vi "Actor Core.vi"(8 "error in":errorcluster, 11 "Main_Control in":refnum<class "Main_Control.lvclass">) -> (0 "error out":errorcluster, 3 "Actor out":refnum<class "Actor.lvclass">)   [LabVIEW 2021, in "Main_Control.lvlib" / "Main_Control.lvclass"]
doc: "(<B>Filename</B>: Actor Framework.lvlib:Actor.lvclass:Actor Core.vi)\n\nReceives messages to the actor, reacts to them, and initiates any error handling that may shut the actor down.\n\nDescendant classes may override this VI to append parallel tasks for the actor to complete while it handles messages. Overrides use the Call Parent Method node."
uses:
  Main_Control.lvclass
  C:/Program Files (x86)/National Instruments/LabVIEW 2021/vi.lib/ActorFramework/Actor/Actor.lvclass
  <vilib>/ActorFramework/Actor/Actor.lvclass
  NI/NI/NI.lvclass
  Camera/Camera/Camera.lvclass
  Utilities/RWC_Actions.ctl
  <vilib>/ActorFramework/Actor/Actor.lvclass/Actor.ctl
  <vilib>/ActorFramework/Message Enqueuer/Message Enqueuer.lvclass/Message Enqueuer.ctl
  Main_Control.lvclass/Main_Control.ctl
  Camera/Camera/Cam task parameters.ctl
  NI/NI/NI task parameters.ctl
  Camera/Camera Messages/Cam prepare task Msg/Cam prepare task Msg.lvclass/Cam prepare task Msg.ctl
  NI/NI Messages/NI prepare task Msg/NI prepare task Msg.lvclass/NI prepare task Msg.ctl
  <vilib>/ActorFramework/Message Enqueuer/Init from Existing Queue.vi
  <vilib>/ActorFramework/Message Enqueuer/Enqueue.vi
  NI/NI Messages/NI start task Msg/NI start task Msg.lvclass
  C:/Program Files (x86)/National Instruments/LabVIEW 2021/vi.lib/ActorFramework/Message/Message.lvclass
  <vilib>/ActorFramework/Stop Msg/Stop Msg.lvclass
  Camera/Camera Messages/Cam prepare task Msg/Cam prepare task Msg.lvclass
  NI/NI Messages/NI prepare task Msg/NI prepare task Msg.lvclass
  NI/NI Messages/NI stop task Msg/NI stop task Msg.lvclass
  <vilib>/ActorFramework/Message Priority Queue/Priority Enqueue.vi
  <vilib>/ActorFramework/Message Enqueuer/Message Enqueuer.lvclass
panel:
  out "time remain":dbl
  in  "Auto":bool
  out "Cam ready":bool
  out "NI ready":bool
  out "Cam":bool
  out "NI":bool
  in  "frame#":dbl=-1.0
  in  "save folder":path=path "D:/zyj workspace/SRIV/Temp File"
  in  "laser option":bool[](array[boolean])=[TRUE, FALSE, TRUE, FALSE]
  in  "buffer page #":dbl=20.0
  in  "flyback line #":dbl=400.0
  in  "camera H":dbl=8.0
  in  "camera W":dbl=768.0
  in  "exposure time":dbl=0.000107 min=1.7e-05 max=10.0
  in  "Update":bool
  in  "Acquire":bool
  out "auto start interval limit":dbl
  out "frame rate":dbl
  in  "laser all on?":bool
  in  "z offset":dbl
  in  "auto interval":dbl
  in  "z scan #":dbl=20.0
  in  "z step size":dbl=0.066
  in  "y pixel size":dbl=0.00059
  in  "y line #":dbl=9600.0
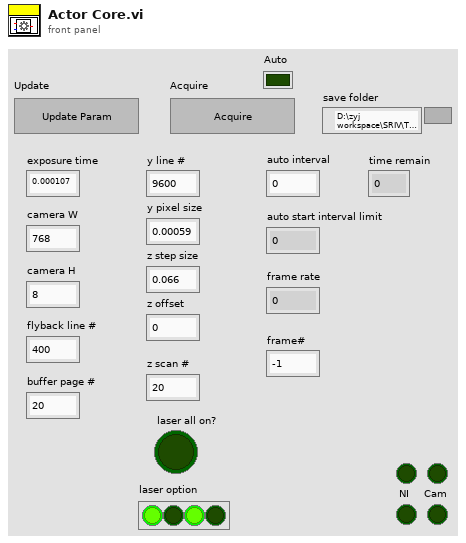
[diagram p1: front panel]
types:
  T1 = typedef "RWC_Actions.ctl" = enum16{"Read", "Write", "Read and Create"}
  T2 = typedef "NI.lvlib/NI.lvclass/NI task parameters.ctl" = cluster{"exposure time":dbl, "camera H":dbl, "y line #":dbl, "flyback line #":dbl, "y pixel size":dbl, "z scan #":dbl, "z step size":dbl, "z offset":dbl, "laser all on?":bool, "laser option":bool[]}
  T3 = typedef "Camera.lvlib/Camera.lvclass/Cam task parameters.ctl" = cluster{"exposure time":dbl, "camera W":dbl, "camera H":dbl, "y line #":dbl, "flyback line #":dbl, "buffer page#":dbl, "frame#":dbl}
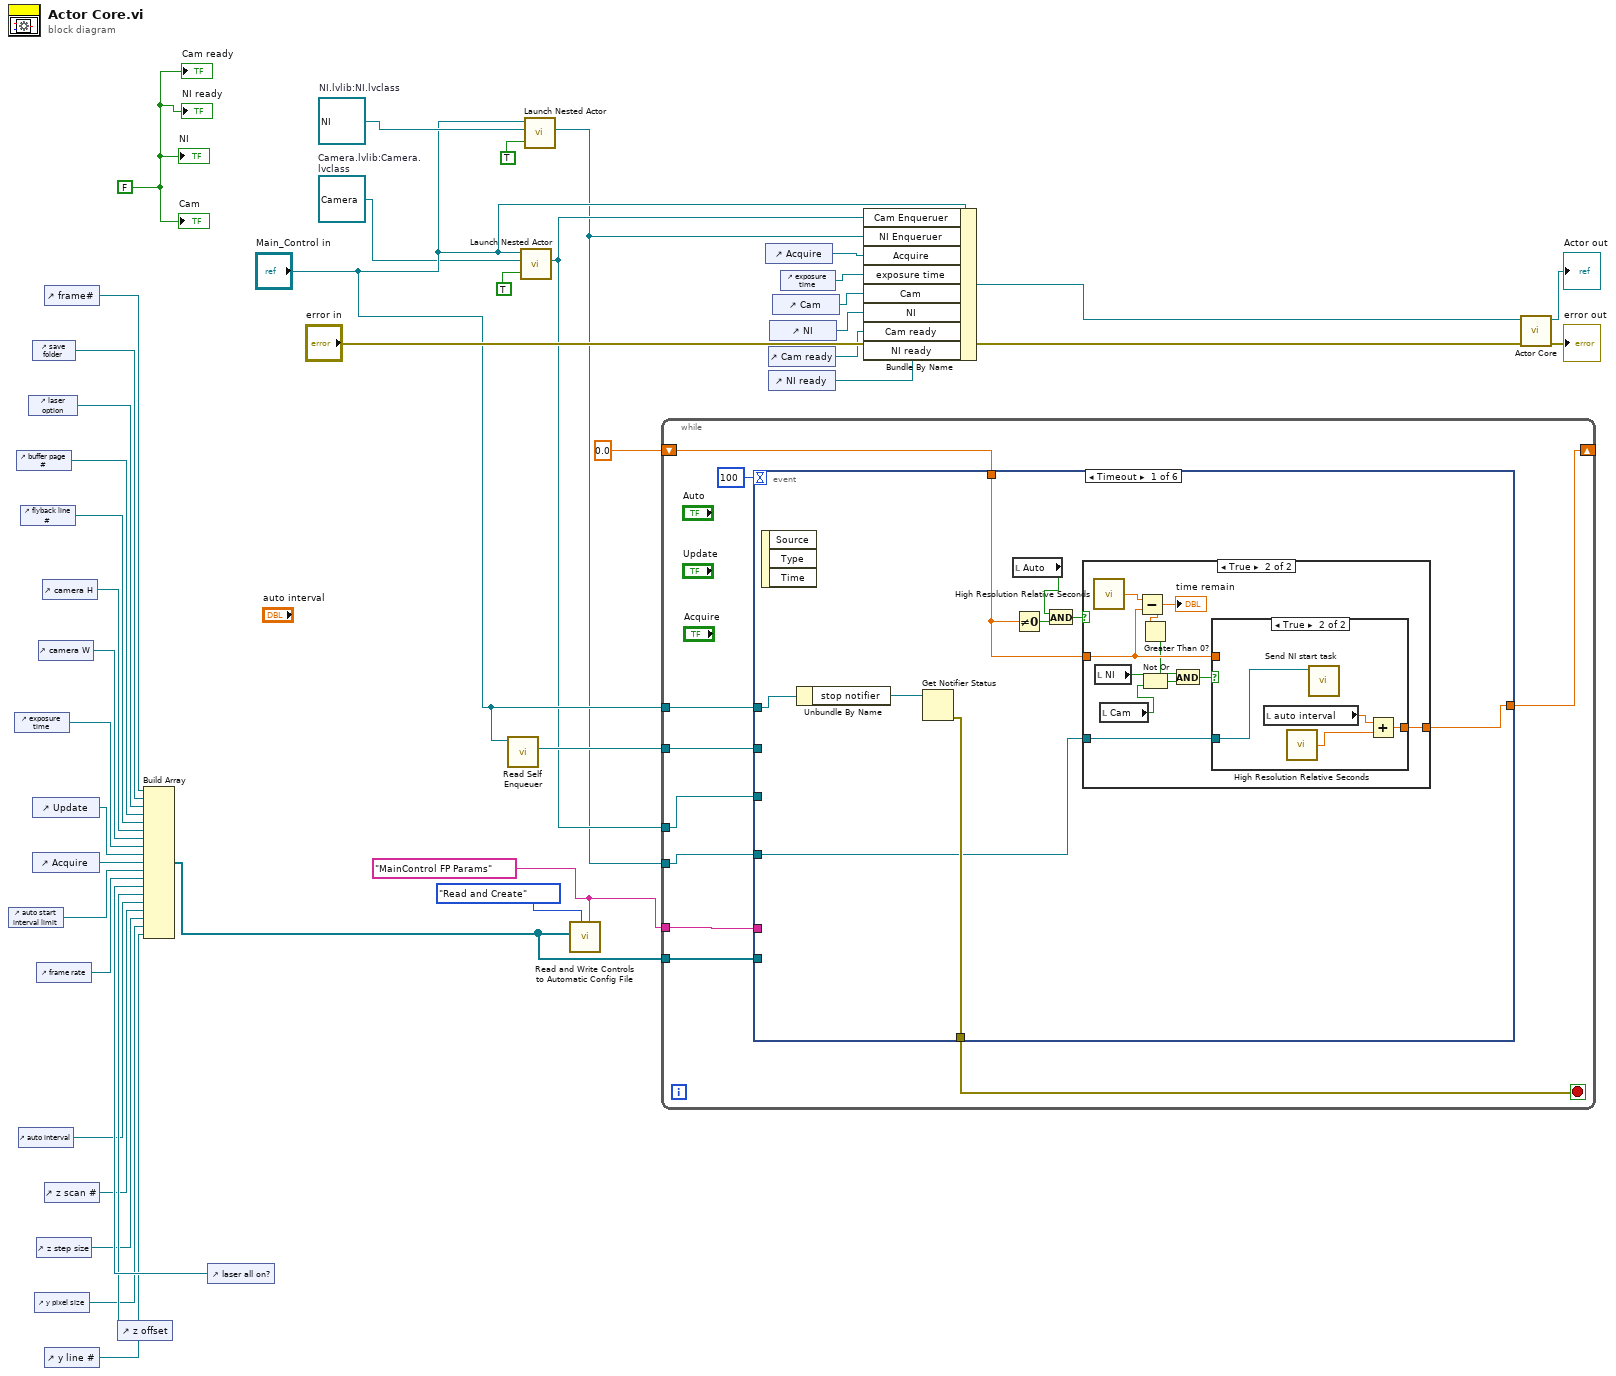
[diagram p0: block diagram]
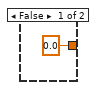
[diagram p2: hidden frame]
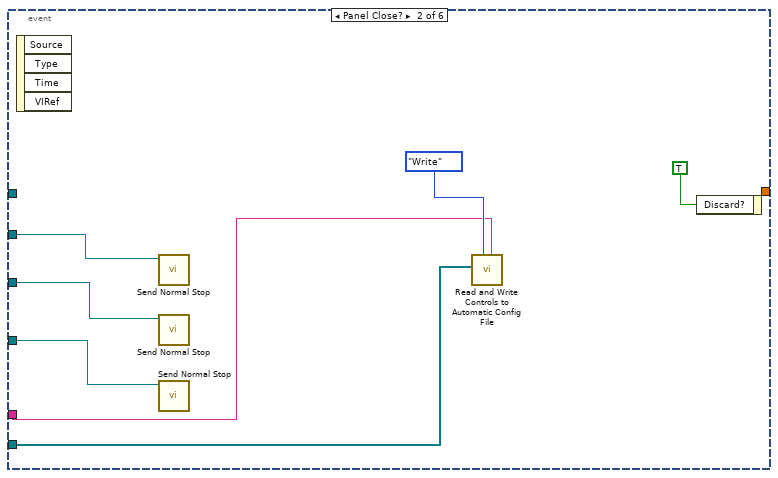
[diagram p4: hidden frame]
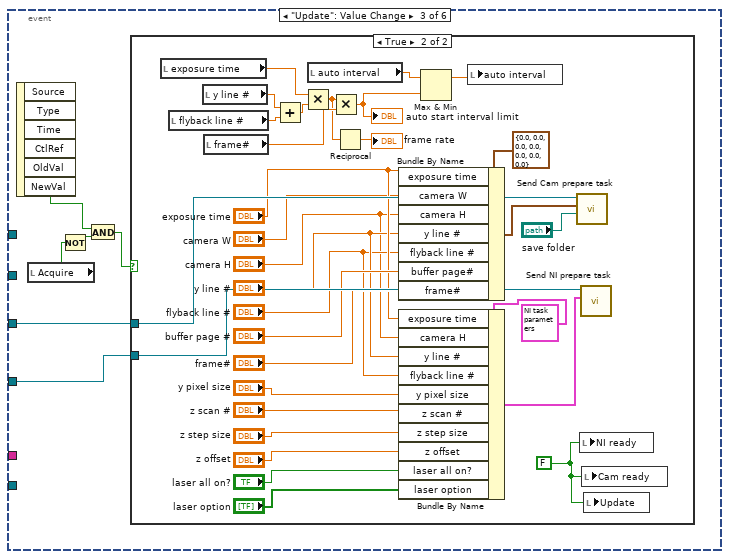
[diagram p5: hidden frame]
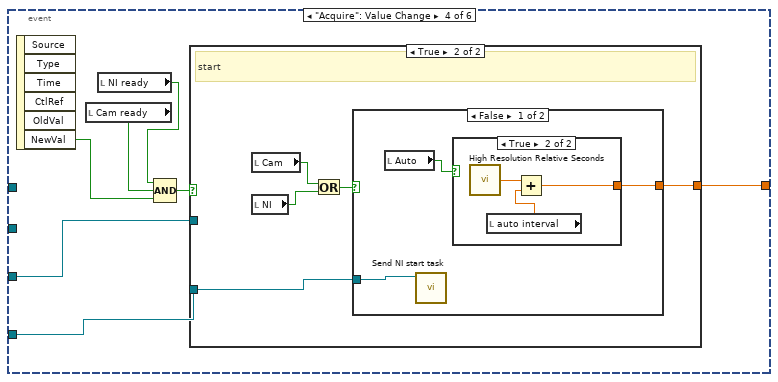
[diagram p7: hidden frame]
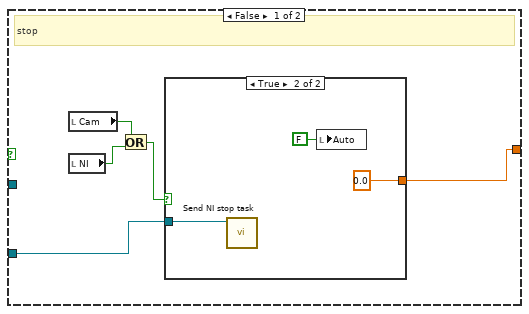
[diagram p8: hidden frame]
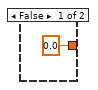
[diagram p10: hidden frame]
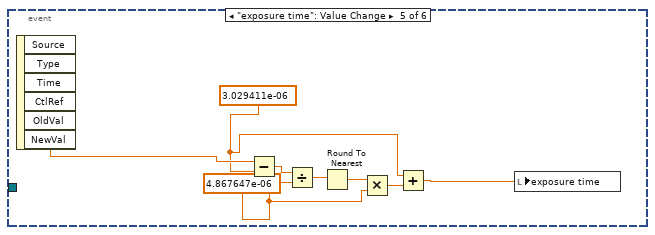
[diagram p12: hidden frame]
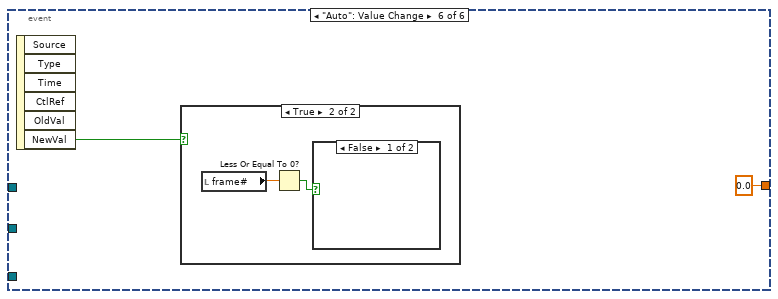
[diagram p13: hidden frame]
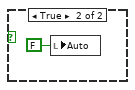
[diagram p15: hidden frame]
diagram:
  w4 = FALSE ("NI")
  w8 = "MainControl FP Params" ("section (optional)")
  w7 = refnum<class "Camera.lvclass"> refnum  # Camera.lvlib:Camera.lvclass
  w38 = refnum<class "NI.lvclass"> refnum  # NI.lvlib:NI.lvclass
  n1 = control-ref of="auto start interval limit"() -> (w18:refnum<vi>)
  n2 = control-ref of="exposure time"() -> (w21:refnum<vi>)
  n3 = control-ref of="buffer page #"() -> (w25:refnum<vi>)
  n4 = control-ref of="auto interval"() -> (w14:refnum<vi>)
  n5 = control-ref of="flyback line #"() -> (w24:refnum<vi>)
  n6 = control-ref of="laser option"() -> (w26:refnum<vi>)
  n7 = control-ref of="save folder"() -> (w27:refnum<vi>)
  n8 = control-ref of="Update"() -> (w20:refnum<vi>)
  n9 = control-ref of="Acquire"() -> (w19:refnum<vi>)
  n10 = control-ref of="y pixel size"() -> (w11:refnum<vi>)
  n11 = control-ref of="frame rate"() -> (w17:refnum<vi>)
  n12 = control-ref of="z step size"() -> (w12:refnum<vi>)
  n13 = control-ref of="camera W"() -> (w22:refnum<vi>)
  n14 = control-ref of="camera H"() -> (w23:refnum<vi>)
  n15 = control-ref of="frame#"() -> (w28:refnum<vi>)
  n16 = control-ref of="z scan #"() -> (w13:refnum<vi>)
  n17 = control-ref of="y line #"() -> (w10:refnum<vi>)
  n18 = control-ref of="z offset"() -> (w15:refnum<vi>)
  n19 = control-ref of="laser all on?"() -> (w16:refnum<vi>)
  n20 = Build Array(w28, w27, w26, w25, w24, w23, w22, w21, w20, w19, w18, w17, w16, w15, w14, w13, w12, w11, w10) -> (w9:refnum<vi>[])
  n21 = call <vilib>:"Read Self Enqueuer.vi"("Actor"="Main_Control in") -> ("Self Enqueuer"=w39:refnum<class "Message Enqueuer.lvclass">)  [unwired: 10 in]
  n22 = call <vilib>:"Launch Nested Actor.vi"("Open Actor Core front panel? (F)"=TRUE, "Nested Actor"=w7, "Caller Actor in"="Main_Control in") -> ("Nested Actor's Enqueuer"=w31:refnum<class "Message Enqueuer.lvclass">)  [unwired: 6 in, 2 out]
  n23 = call <vilib>:"Launch Nested Actor.vi"("Open Actor Core front panel? (F)"=TRUE, "Nested Actor"=w38, "Caller Actor in"="Main_Control in") -> ("Nested Actor's Enqueuer"=w30:refnum<class "Message Enqueuer.lvclass">)  [unwired: 6 in, 2 out]
  n24 = call "Read and Write Controls to Automatic Config File.vi"("file name"=w8, "Action"=RWC_Actions."Read and Create", "Control References"=w9) -> ()  [unwired: 8 in, 1 out]
  n25 = while {
    tunnel: "Main_Control in" -> [w51]
    tunnel: w39 -> [w49]
    tunnel: w31 -> [w48]
    tunnel: w30 -> [w47]
    tunnel: w9 -> [w46]
    tunnel: w8 -> [w45]
    shift-right: [w44] -> _
    shift-left: 0.0 ("relative seconds") -> [w43]
    stop <- w50 stop-if-true
    n26 = event shown="[0] Timeout" {
      selector: _ -> [_ _ _ _ _ _]
      dyn-events: _ -> [_ _ _ _ _ _]
      timeout: 100 -> [_ _ _ _ _ _]
      tunnel: w51 -> [w61 _ _ _ _ _]
      tunnel: [w59 _ _ _ _ _] -> w50
      tunnel: w49 -> [_ w84 _ _ _ _]
      tunnel: w48 -> [_ w83 w89 w127 _ _]
      tunnel: w47 -> [w54 w82 w90 w128 _ _]
      tunnel: w46 -> [_ w79 _ _ _ _]
      tunnel: w45 -> [_ w78 _ _ _ _]
      tunnel: [w53 _ _ w122 _ 0.0 ("relative seconds")] -> w44
      tunnel: w43 -> [w55 _ _ _ _ _]
      event Timeout {
        n27 = event-data() -> ()  [unwired: 1 in, 3 out]
        n28 = Unbundle By Name(w61) -> ("stop notifier"=w60:refnum<notifier>)
        n29 = Get Notifier Status(notifier=w60) -> (error out=w59:errorcluster)  [unwired: 1 in, 4 out]
        n30 = local read "Auto"() -> (w56:bool)
        n31 = Not Equal To 0?(x=w55) -> (x != 0?=w57:bool)
        n32 = And(x=w56, y=w57) -> (x .and. y?=w58:bool)
        n33 = case shown="True" w58 {
          tunnel: w55 -> [_ w64]
          tunnel: w54 -> [_ w72]
          tunnel: [0.0 ("relative seconds") w67] -> w53
          frame False {
          }
          frame True {
            n34 = call <vilib>:"High Resolution Relative Seconds.vi"() -> ("relative seconds"=w65:dbl)
            n35 = local read "NI"() -> (w68:bool)
            n36 = local read "Cam"() -> (w69:bool)
            n37 = Subtract(x=w65, y=w64) -> (x-y=w66:dbl)
            "time remain" <- w66
            n38 = Greater Than 0?(x=w66) -> (x > 0?=w63:bool)
            n39 = Not Or(1:w69, 2:w68) -> (0:w70:bool)
            n40 = And(x=w63, y=w70) -> (x .and. y?=w71:bool)
            n41 = case shown="True" w71 {
              tunnel: w72 -> [_ w77]
              tunnel: w64 -> [w73 _]
              tunnel: [w73 w74] -> w67
              frame False {
              }
              frame True {
                n42 = local read "auto interval"() -> (w76:dbl)
                n43 = call <vilib>:"High Resolution Relative Seconds.vi"() -> ("relative seconds"=w75:dbl)
                n44 = call "Send NI start task.vi"("Message Enqueuer"=w77) -> ()  [unwired: 9 in, 2 out]
                n45 = Add(x=w76, y=w75) -> (x+y=w74:dbl)
              }
            }
          }
        }
      }
      event Panel Close? {
        n46 = event-data() -> ()  [unwired: 1 in, 4 out]
        n47 = call <vilib>:"Send Normal Stop.vi"("Message Enqueuer"=w84) -> ()  [unwired: 10 in, 1 out]
        n48 = call <vilib>:"Send Normal Stop.vi"("Message Enqueuer"=w83) -> ()  [unwired: 10 in, 1 out]
        n49 = call <vilib>:"Send Normal Stop.vi"("Message Enqueuer"=w82) -> ()  [unwired: 10 in, 1 out]
        n50 = call "Read and Write Controls to Automatic Config File.vi"("file name"=w78, "Action"=RWC_Actions."Write", "Control References"=w79) -> ()  [unwired: 8 in, 1 out]
        n51 = event-data("Discard?"=TRUE) -> ()  [unwired: 1 in, 1 out]
      }
      event "Update": Value Change {
        n52 = event-data() -> ("NewVal"=w88:bool)  [unwired: 1 in, 5 out]
        n53 = local read "Acquire"() -> (w85:bool)
        n54 = Not(x=w85) -> (.not. x?=w86:bool)
        n55 = And(x=w88, y=w86) -> (x .and. y?=w87:bool)
        n56 = case shown="True" w87 {
          tunnel: w90 -> [_ w121]
          tunnel: w89 -> [_ w120]
          frame False {
          }
          frame True {
            w102 = FALSE ("NI ready")
            n57 = local read "exposure time"() -> (w95:dbl)
            n58 = local read "flyback line #"() -> (w99:dbl)
            n59 = local read "y line #"() -> (w100:dbl)
            n60 = local read "frame#"() -> (w94:dbl)
            n61 = Add(x=w100, y=w99) -> (x+y=w96:dbl)
            n62 = Multiply(x=w95, y=w96) -> (x*y=w92:dbl)
            n63 = local read "auto interval"() -> (w98:dbl)
            n64 = Multiply(x=w92, y=w94) -> (x*y=w93:dbl)
            "auto start interval limit" <- w93
            n65 = Reciprocal(x=w92) -> (1/x=→"frame rate":dbl)
            n66 = Bundle By Name(cluster=T3 {"exposure time"=0.0, "camera W"=0.0, "camera H"=0.0, "y line #"=0.0, "flyback line #"=0.0, "buffer page#"=0.0, "frame#"=0.0} ("Cam task parameters"), "exposure time"="exposure time", "camera W"="camera W", "camera H"="camera H", "y line #"="y line #", "flyback line #"="flyback line #", "buffer page#"="buffer page #", "frame#"="frame#") -> (w118:T3)
            n67 = Bundle By Name(cluster=T2 {"exposure time"=0.0, "camera H"=0.0, "y line #"=0.0, "flyback line #"=0.0, "y pixel size"=0.0, "z scan #"=0.0, "z step size"=0.0, "z offset"=0.0, "laser all on?"=FALSE, "laser option"=[]} ("NI task parameters"), "exposure time"="exposure time", "camera H"="camera H", "y line #"="y line #", "flyback line #"="flyback line #", "y pixel size"="y pixel size", "z scan #"="z scan #", "z step size"="z step size", "z offset"="z offset", "laser all on?"="laser all on?", "laser option"="laser option") -> (w116:T2)
            n68 = Max & Min(x=w98, y=w93) -> (max(x,y)=w97:dbl)  [unwired: 1 out]
            n69 = local write "auto interval"(w97) -> ()
            n70 = call "Send Cam prepare task.vi"("save folder"="save folder", "Cam task parameters"=w118, "Message Enqueuer"=w120) -> ()  [unwired: 7 in, 2 out]
            n71 = local write "NI ready"(w102) -> ()
            n72 = call "Send NI prepare task.vi"("NI task parameters"=w116, "Message Enqueuer"=w121) -> ()  [unwired: 8 in, 2 out]
            n73 = local write "Cam ready"(w102) -> ()
            n74 = local write "Update"(w102) -> ()
          }
        }
      }
      event "Acquire": Value Change {
        n75 = event-data() -> ("NewVal"=w124:bool)  [unwired: 1 in, 5 out]
        n76 = local read "Cam ready"() -> (w125:bool)
        n77 = local read "NI ready"() -> (w126:bool)
        n78 = Compound Arithmetic op=AND(w126, w125, w124) -> (w123:bool)
        n79 = case shown="True" w123 {
          tunnel: w128 -> [w133 w141]
          tunnel: w127 -> [_ _]
          tunnel: [w129 w137] -> w122
          frame False {
            # "stop"
            n80 = local read "Cam"() -> (w132:bool)
            n81 = local read "NI"() -> (w131:bool)
            n82 = Or(x=w132, y=w131) -> (x .or. y?=w130:bool)
            n83 = case shown="True" w130 {
              tunnel: w133 -> [_ w136]
              tunnel: [_ 0.0] -> w129
              frame False {
              }
              frame True {
                n84 = call "Send NI stop task.vi"("Message Enqueuer"=w136) -> ()  [unwired: 9 in, 2 out]
                n85 = local write "Auto"(FALSE ("Auto")) -> ()
              }
            }
          }
          frame True {
            # "start"
            n86 = local read "Cam"() -> (w140:bool)
            n87 = local read "NI"() -> (w139:bool)
            n88 = Or(x=w140, y=w139) -> (x .or. y?=w138:bool)
            n89 = case shown="False" w138 {
              tunnel: w141 -> [w144 _]
              tunnel: [w142 _] -> w137
              frame False {
                n90 = local read "Auto"() -> (w143:bool)
                n91 = call "Send NI start task.vi"("Message Enqueuer"=w144) -> ()  [unwired: 9 in, 2 out]
                n92 = case shown="True" w143 {
                  tunnel: [0.0 w146] -> w142
                  frame False {
                  }
                  frame True {
                    n93 = call <vilib>:"High Resolution Relative Seconds.vi"() -> ("relative seconds"=w148:dbl)
                    n94 = local read "auto interval"() -> (w147:dbl)
                    n95 = Add(x=w148, y=w147) -> (x+y=w146:dbl)
                  }
                }
              }
              frame True {
              }
            }
          }
        }
      }
      event "exposure time": Value Change {
        w152 = 4.867647e-06 ("y")
        w150 = 3.029411e-06 ("y")
        n96 = event-data() -> ("NewVal"=w156:dbl)  [unwired: 1 in, 5 out]
        n97 = Subtract(x=w156, y=w150) -> (x-y=w155:dbl)
        n98 = Divide(x=w155, y=w152) -> (x/y=w154:dbl)
        n99 = Round To Nearest(number=w154) -> (nearest integer value=w153:dbl)
        n100 = Multiply(x=w153, y=w152) -> (x*y=w151:dbl)
        n101 = Add(x=w150, y=w151) -> (x+y=w149:dbl)
        n102 = local write "exposure time"(w149) -> ()
      }
      event "Auto": Value Change {
        n103 = event-data() -> ("NewVal"=w158:bool)  [unwired: 1 in, 5 out]
        n104 = case shown="True" w158 {
          frame False {
          }
          frame True {
            n105 = local read "frame#"() -> (w160:dbl)
            n106 = Less Or Equal To 0?(x=w160) -> (x <= 0?=w159:bool)
            n107 = case shown="False" w159 {
              frame False {
              }
              frame True {
                n108 = local write "Auto"(FALSE ("Auto")) -> ()
              }
            }
          }
        }
      }
    }
  }
  n109 = control-ref of="Acquire"() -> (w33:refnum<vi>)
  n110 = control-ref of="Cam ready"() -> (w3:refnum<vi>)
  n111 = control-ref of="NI ready"() -> (w2:refnum<vi>)
  n112 = control-ref of="NI"() -> (w5:refnum<vi>)
  n113 = control-ref of="Cam"() -> (w6:refnum<vi>)
  n114 = control-ref of="exposure time"() -> (w32:refnum<vi>)
  n115 = Bundle By Name(cluster="Main_Control in", "Cam Enqueruer"=w31, "NI Enqueruer"=w30, "Acquire"=w33, "exposure time"=w32, "Cam"=w6, "NI"=w5, "Cam ready"=w3, "NI ready"=w2) -> (w34:refnum<class "Main_Control.lvclass">)
  n116 = call-parent "Actor Core.vi"("error in"="error in", "Actor in"=w34) -> ("error out"=→"error out":errorcluster, "Actor out"=→"Actor out":refnum<class "Actor.lvclass">)  [unwired: 8 in]
  "NI" <- w4
  "Cam" <- w4
  "NI ready" <- w4
  "Cam ready" <- w4
